vi "Parse updateUser.vi"(8 "error in (no error)":errorcluster, 11 "JSON (UTF-8) String":string) -> (0 "error out":errorcluster, 2 "Telegram State":T1, 3 "Variant":variant)   [LabVIEW 2015, in "JSON Library.lvlib"]
doc: "Created IvanLis by LabVIEW Portal\nProfile: http://labviewportal.org/memberlist.php?mode=viewprofile&u=987\neMail: IvanLisanov@gMail.com\nTelegram: https://t.me/IvanLis"
uses:
  JSON Library.lvlib
  Telegram Library/TypeDef/Telegram State.ctl
  TypeDef/User.ctl
  Telegram Library/Telegram Library.lvlib
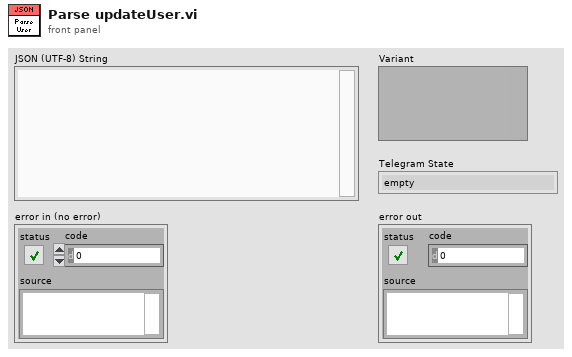
[diagram p1: front panel]
types:
  T1 = typedef "Telegram Library.lvlib/Telegram State.ctl" = enum16{"empty", "ok", "authorizationStateClosed", "authorizationStateWaitTdlibParameters", "authorizationStateWaitEncryptionKey", "authorizationStateWaitPhoneNumber", "authorizationStateWaitCode", "connectionStateWaitingForNetwork", "connectionStateConnectingToProxy", "connectionStateUpdating", "connectionStateConnecting", "connectionStateReady", "updateUser_user", "updateNewChat_chat", "updateNewMessage_Text", "updateChatLastMessage_Text", "updateDeleteMessages", "updateChatPosition", "ChatHistoryMessages_Text"}
  T2 = typedef "JSON Library.lvlib/user.ctl" = cluster{"@type":string, "id":i64, "first_name":string, "last_name":string, "username":string, "phone_number":string}
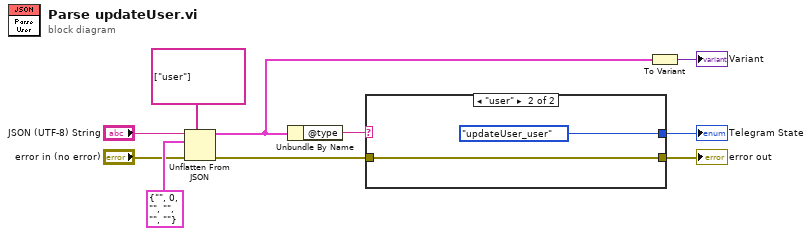
[diagram p0: block diagram]
diagram:
  n1 = Unflatten From JSON(path=string[] ["user"], JSON string="JSON (UTF-8) String", type and defaults=T2 {"@type"="", "id"=0, "first_name"="", "last_name"="", "username"="", "phone_number"=""} ("user"), error in (no error)="error in (no error)") -> (value=w7:T2, error out=w6:errorcluster)  [unwired: 3 in]
  n2 = Unbundle By Name(w7) -> ("@type"=w5:string)
  n3 = case shown="\"user\"" w5 {
    tunnel: w6 -> [w11 w12]
    tunnel: [w11 w12] -> w1
    tunnel: [_ Telegram_State."updateUser_user" ("Telegram State")] -> w2
    frame Default {
    }
    frame "user" {
    }
  }
  "Telegram State" <- w2
  "error out" <- w1
  n4 = To Variant(anything=w7) -> (Variant=→"Variant":variant)
